vi "XLP80_Action_InitDebug.vi"(8 "err in":errorcluster) -> (0 "err out":errorcluster, 2 "Debug OUT":T1)   [LabVIEW 2021]
uses:
  XLP80_FGlob/1886_FGlob_TDefs_Enum_FGlobItems.ctl
  XLP80_General_Libs/Kirschenhofer_Libs/KH Turck EthernetIP 17.12/KH TURCK TypeDefs FGlob.ctl
  XLP80_Globals/Globals_Settings_XLP80.vi
  XLP80_Globals/XLP80_Globals_Status.vi
  XLP80_Globals/XLP80_Globals_Action.vi
panel:
  out "Debug_AI Names":string[](array[string])=["Fp_HPRU_TS1", "Fp_HPRU_TS2", "Fp_So_TS", "AT_EXH_TS", "EU_DCDCi_TS", "EI_DCDC24V_TS", "EI_DIV25A_TS", "EI_DCDC12V_TS", "EI_ETC_TS", "EI_DIV40A_TS", "EI_DCDCi_TS", "EI_DCDCo_TS", "EI_BAT_TS", "EI_LOAD_TS", "Reserve_AI_4_2", "Reserve_AI_4_3", "AT_Si_TS", "AT_So_TS", "CT_Si_TS", "CT_So_TS", "Ck_CP1i_TS", "Cp_CP1i_TS", "Cp_CP1o_TS", "Cp_CP2o_TS"]
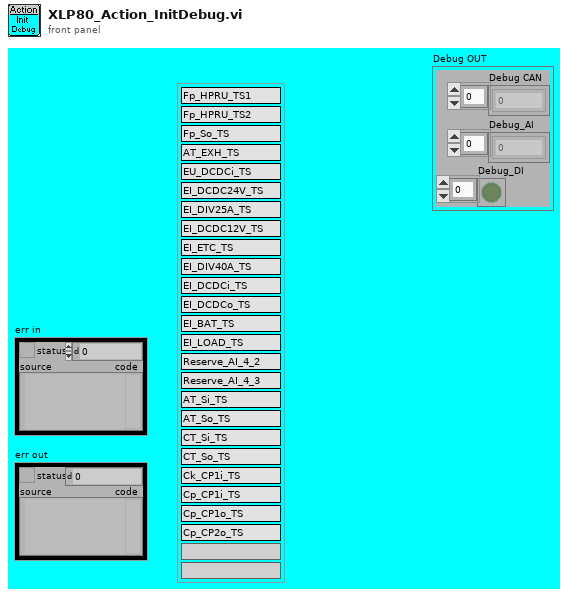
[diagram p1: front panel]
types:
  T1 = cluster{"Debug CAN":dbl[], "Debug_AI":sgl[], "Debug_DI":bool[]}
  T2 = typedef "XLP80_Action_TDefEnumControl.ctl" = enum16{"Testmode_A", "Testmode_B"}
  T3 = typedef "KH_DAQ_TypeDefs_Cluster AI.ctl" = cluster{"Signal Name":string[], "Description":string[], "Phys Unit":string[], "Messbereich":T4[], "Chan":u16[], "Phys Min":sgl[], "Phys Max":sgl[], "Offset":sgl[], "Nr":u16[], "SensorType 2":T5[], "Bereich":T6[]}
  T4 = typedef "KH_DAQ_TypeDefs_Messbereich.ctl" = enum16{"-10V ... +10V", "0V ... +10V", "+2V ... +10V", "0V ... +5V", "+1V ... +5V", "-1V ... +1V", "-500mV ... +500mV", "-100mV ... +100mV", "-50mV ... +50mV", "0mA ... +20mA", "+4mA ... +20mA", "-20mA ... +20mA", "0 Ohm ... 100 Ohm", "0 Ohm ... 400 Ohm", "0 Ohm ... 2000 Ohm", "0 Ohm ... 4000 Ohm", "-200°C ... 150°C PT100", "-200°C ... 150°C PT200", "-200°C ... 150°C PT500", "-200°C ... 150°C PT1000", "-60°C ... 150°C Ni100", "-60°C ... 150°C Ni1000", "-200°C ... 850°C PT100", "-200°C ... 850°C PT200", "-200°C ... 850°C PT500", "-200°C ... 850°C PT1000", "-50°C ... 250°C Ni100", "-50°C ... 250° Ni 1000"}
  T5 = typedef "KH EthernetIPConfig TypeDefs ModuleTyp.ctl" = enum16{"TBEN-S2-4AI", "TBEN-S1-8DXP", "TBEN-S2-2RFID-4DXP", "TBEN-S2-4AO", "TBEN-S2-4IOL"}
  T6 = typedef "KH_DAQ_TypeDefs_Bereich.ctl" = enum16{"Standard", "extended Range", "NE43", ""}
  T7 = typedef "KH_DAQ_TURCK_TypeDefs_Cluster DI.ctl" = cluster{"Signal Name":string[], "Description":string[], "Chan":u16[], "Inv":bool[], "Nr":u16[], "SensorType":T5[]}
  T8 = cluster{"Signal Name":string[], "Description":string[], "Unit":string[], "Min":dbl[], "Max":dbl[], "HV & Software":bool[], "Basis Funktion":bool[], "Power Management":bool[], "OperationMode":bool[], "Shutdown":bool[], "Alarm":bool[], "LogEnable":bool[]}
  T9 = cluster{"Signal Name":string[], "Description":string[], "Unit":string[], "Min":dbl[], "Max":dbl[], "TestmodeA":bool[], "LogEnable":bool[]}
  T10 = typedef "KH TURCK TypeDefs FGlob.ctl" = enum16{"Put one", "Put all", "Recall one", "Recall all"}
  T11 = typedef "1886_FGlob_TDefs_Enum_FGlobItems.ctl" = enum16{"Put one", "Put all", "Recall one", "Recall all"}
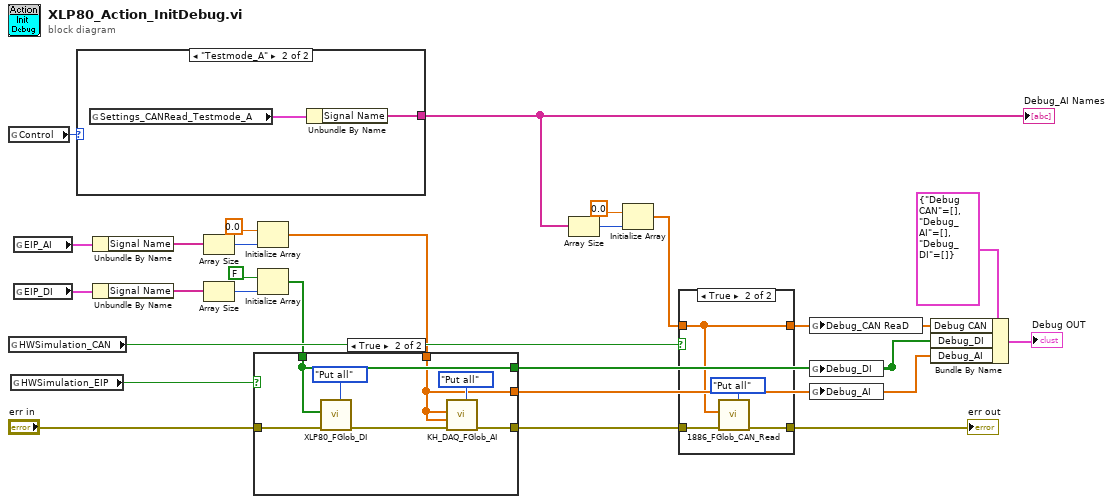
[diagram p0: block diagram]
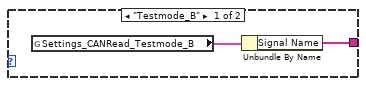
[diagram p3: hidden frame]
diagram:
  n1 = global read "XLP80_Globals_Status.vi" "Control"() -> (w20:T2)
  n2 = global read "Globals_Settings_XLP80.vi" "HWSimulation_CAN"() -> (w25:bool)
  n3 = global read "Globals_Settings_XLP80.vi" "HWSimulation_EIP"() -> (w12:bool)
  n4 = global read "Globals_Settings_XLP80.vi" "EIP_AI"() -> (w15:T3)
  n5 = global read "Globals_Settings_XLP80.vi" "EIP_DI"() -> (w5:T7)
  n6 = case shown="\"Testmode_A\"" w20 {
    tunnel: [w26 w28] -> w16
    frame "Testmode_B" {
      n7 = global read "Globals_Settings_XLP80.vi" "Settings_CANRead_Testmode_B"() -> (w27:T8)
      n8 = Unbundle By Name(w27) -> ("Signal Name"=w26:string[])
    }
    frame "Testmode_A" {
      n9 = global read "Globals_Settings_XLP80.vi" "Settings_CANRead_Testmode_A"() -> (w29:T9)
      n10 = Unbundle By Name(w29) -> ("Signal Name"=w28:string[])
    }
  }
  "Debug_AI Names" <- w16
  n11 = Unbundle By Name(w15) -> ("Signal Name"=w9:string[])
  n12 = Unbundle By Name(w5) -> ("Signal Name"=w8:string[])
  n13 = Array Size(array=w9) -> (size(s)=w10:i32)
  n14 = Array Size(array=w8) -> (size(s)=w7:i32)
  n15 = Initialize Array(sgl 0.0 ("Numeric"), w10) -> (w2:sgl[])
  n16 = Initialize Array(FALSE, w7) -> (w4:bool[])
  n17 = case shown="True" w12 {
    tunnel: "err in" -> [w31 w39]
    tunnel: [w31 w35] -> w13
    tunnel: w4 -> [w32 w37]
    tunnel: [w32 w37] -> w3
    tunnel: w2 -> [w30 w33]
    tunnel: [w30 w33] -> w1
    frame False {
    }
    frame True {
      n18 = call "XLP80_FGlob_DI.vi"("Function (Recall One)"=1886_FGlob_TDefs_Enum_FGlobItems."Put all", "err in"=w39, "DI Values IN"=w37) -> ("err out"=w36:errorcluster)  [unwired: 6 in, 2 out]
      n19 = call "KH_DAQ_FGlob_AI.vi"("Function (Recall One)"=KH_TURCK_TypeDefs_FGlob."Put all", "err in"=w36, "AI Unscaled IN"=w33, "AI Values IN"=w33) -> ("err out"=w35:errorcluster)  [unwired: 4 in, 3 out]
    }
  }
  n20 = Array Size(array=w16) -> (size(s)=w19:i32)
  n21 = Initialize Array(0.0 ("Numeric"), w19) -> (w17:dbl[])
  n22 = case shown="True" w25 {
    tunnel: w13 -> [w41 w44]
    tunnel: [w41 w43] -> w21
    tunnel: w17 -> [w40 w42]
    tunnel: [w40 w42] -> w24
    frame False {
    }
    frame True {
      n23 = call "1886_FGlob_CAN_Read.vi"("Function (Recall One)"=1886_FGlob_TDefs_Enum_FGlobItems."Put all", "err in"=w44, "AI Values IN"=w42) -> ("err out"=w43:errorcluster)  [unwired: 6 in, 2 out]
    }
  }
  "err out" <- w21
  n24 = global write "XLP80_Globals_Action.vi" "Debug_CAN ReaD"(w24) -> ()
  n25 = global write "XLP80_Globals_Action.vi" "Debug_DI"(w3) -> ()
  n26 = global write "XLP80_Globals_Action.vi" "Debug_AI"(w1) -> ()
  n27 = Bundle By Name(cluster=T1 {"Debug CAN"=[], "Debug_AI"=[], "Debug_DI"=[]} ("Debug OUT"), "Debug CAN"=w24, "Debug_DI"=w3, "Debug_AI"=w1) -> (→"Debug OUT":T1)
